vi "Test Config Migration.vi"() -> ()   [LabVIEW 2023]
panel:
  out "error out":errorcluster
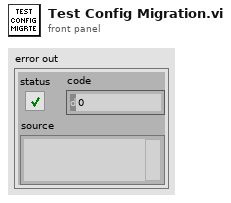
[diagram p1: front panel]
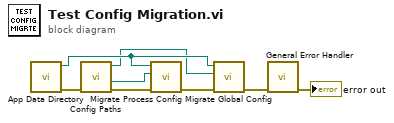
[diagram p0: block diagram]
diagram:
  n1 = call "App Data Directory.vi"() -> ("error out"=w8:errorcluster, "App Data Directory"=w4:path)  [unwired: 10 in]
  n2 = call "Config Paths.vi"("error in (no error)"=w8) -> ("error out"=w7:errorcluster, "Process Config"=w6:path, "Global Config"=w3:path)  [unwired: 8 in]
  n3 = call "Migrate Process Config.vi"("error in (no error)"=w7, "Old Process Config"=w6, "App Data Directory"=w4) -> ("error out"=w5:errorcluster)  [unwired: 8 in]
  n4 = call "Migrate Global Config.vi"("error in (no error)"=w5, "Old Global Config"=w3, "App Data Directory"=w4) -> ("error out"=w2:errorcluster)  [unwired: 8 in]
  n5 = call <vilib>:"General Error Handler.vi"("error in (no error)"=w2) -> ("error out"=→"error out":errorcluster)  [unwired: 10 in, 4 out]
